vi "CT_MagPWMCurrent.vi"(8 "Magnet Pulse Timing":dbl(slide) min=-7.0 max=0.0 scale format="%.3f", 11 "Coil Currents":waveform(dbl)[](graph)=[{"t0"=timestamp(3383307443.4356585 s since 1904-01-01), "dt"=0.0033333, "Y"=array[1000 elements], "attributes"=variant("NI_ChannelName"=variant(string "Current_CoilC"), "NI_UnitDescription"=variant(string "Volts"))}, {"t0"=timestamp(3383307443.4356723 s since 1904-01-01), "dt"=0.0033333, "Y"=array[1000 elements], "attributes"=variant("NI_ChannelName"=variant(string "Current_CoilB"), "NI_UnitDescription"=variant(string "Volts"))}, {"t0"=timestamp(3383307443.4356866 s since 1904-01-01), "dt"=0.0033333, "Y"=array[1000 elements], "attributes"=variant("NI_ChannelName"=variant(string "Current_CoilA"), "NI_UnitDescription"=variant(string "Volts"))}]) -> (3 "Mag Current and Names Out":T1(array[cluster])=[{"Coil Current"=-0.10198014417279211, "Coil Name"="CoilC"}, {"Coil Current"=-0.13102222106781625, "Coil Name"="CoilD"}, {"Coil Current"=36.48458663452108, "Coil Name"="CoilE"}])   [LabVIEW 2016]
uses:
  <vilib>/Analysis/baseanly.llb/Mean (DBL).vi
  <vilib>/Analysis/NI_AALBase.lvlib
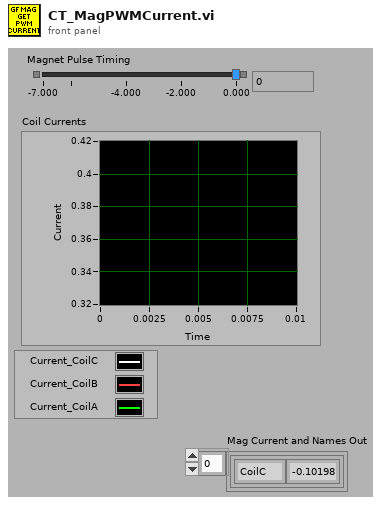
[diagram p1: front panel]
types:
  T1 = cluster{"Coil Current":dbl, "Coil Name":string}[]
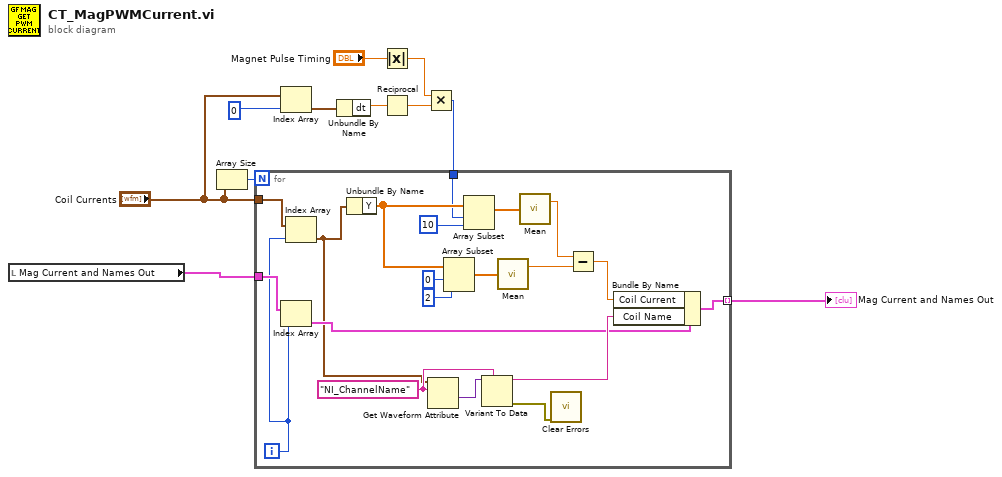
[diagram p0: block diagram]
diagram:
  n1 = local read "Mag Current and Names Out"() -> (w3:T1)
  n2 = Array Size(array="Coil Currents") -> (size(s)=w1:i32)
  n3 = Index Array(array="Coil Currents", index=0) -> (element=w11:waveform(dbl))
  n4 = Unbundle By Name(w11) -> ("dt"=w10:dbl)
  n5 = Absolute Value(x="Magnet Pulse Timing") -> (abs(x)=w6:dbl)
  n6 = Reciprocal(x=w10) -> (1/x=w7:dbl)
  n7 = Multiply(x=w6, y=w7) -> (x*y=w5:i32)
  n8 = for {
    N: w1 -> [_]
    tunnel: "Coil Currents" -> [w13]
    tunnel: w5 -> [w26]
    tunnel: w3 -> [w16]
    tunnel: [w22] -> w4 mode=indexing
    i -> [w14]
    w18 = "NI_ChannelName" ("name")
    n9 = Index Array(array=w16, index=w14) -> (element=w15:cluster{"Coil Current":dbl, "Coil Name":string})
    n10 = Index Array(array=w13, index=w14) -> (element=w12:waveform(dbl))
    n11 = Unbundle By Name(w12) -> ("Y"=w27:dbl[])
    n12 = Get Waveform Attribute(6:w18, 7:w12) -> (1:w20:variant)  [unwired: 2 in, 3 out]
    n13 = Array Subset(array=w27, index=0, length=2) -> (w29:dbl[])
    n14 = Array Subset(array=w27, index=w26, length=10) -> (w24:dbl[])
    n15 = Variant To Data(type=w18, Variant=w20) -> (data=w17:string, error out=w19:errorcluster)  [unwired: 1 in]
    n16 = call-poly <vilib>:"Mean.vi"("X"=w29) -> ("mean"=w28:dbl)  [unwired: 1 out]
    n17 = call-poly <vilib>:"Mean.vi"("X"=w24) -> ("mean"=w23:dbl)  [unwired: 1 out]
    n18 = call <vilib>:"Clear Errors.vi"("error in (no error)"=w19) -> ()  [unwired: 5 in, 2 out]
    n19 = Subtract(x=w23, y=w28) -> (x-y=w21:dbl)
    n20 = Bundle By Name(cluster=w15, "Coil Current"=w21, "Coil Name"=w17) -> (w22:cluster{"Coil Current":dbl, "Coil Name":string})
  }
  "Mag Current and Names Out" <- w4
